vi "FPGA_Array to XY.vi"(7 "Init":bool, 11 "All Random Array":fxp<+/-,32,16>[](array[numeric])) -> (0 "y offset new":i16, 1 "y amp. new":fxp<+,16,0>, 2 "x offset new":i16, 3 "x amp. new":fxp<+,16,0>)   [LabVIEW 2015]
uses:
  Controls/FPGA_Array to XYAO State.ctl
  <vilib>/rvi/Emulation/niFpgaGetClockAttributes.vi
  <vilib>/rvi/Emulation/niFpgaSctlEmulationGetInTimedLoop.vi
  <vilib>/rvi/Emulation/niFpgaEmulationReportErrorSimple.vi
  <vilib>/rvi/Emulation/niFpgaCriticalErrorInLSC.vi
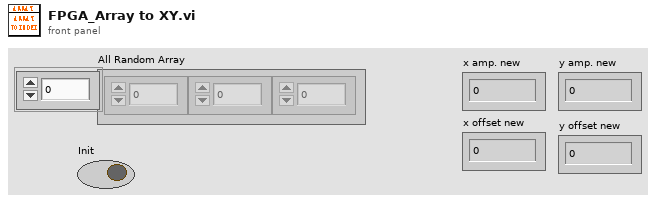
[diagram p1: front panel]
types:
  T1 = typedef "FPGA_Array to XYAO State.ctl" = enum16{"Initial", "Output"}
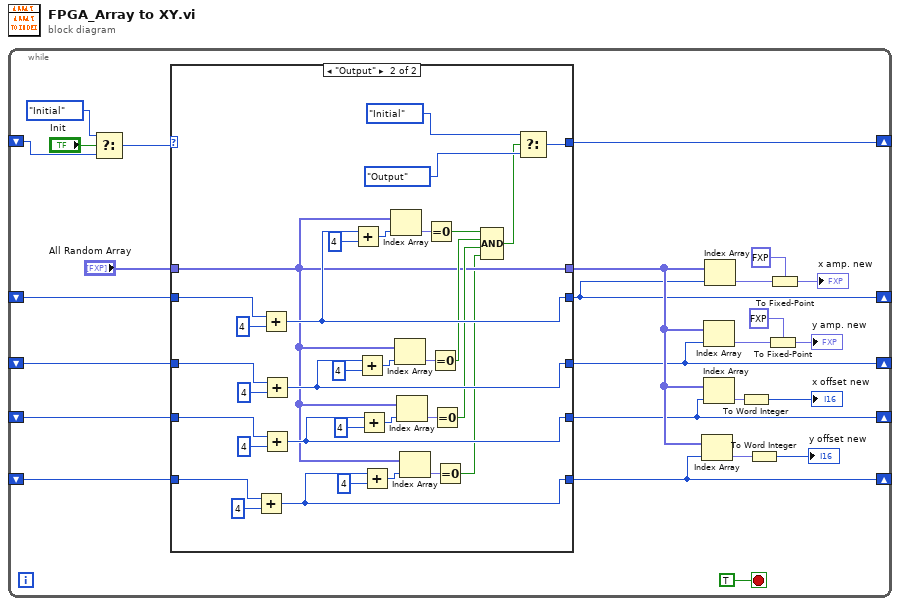
[diagram p0: block diagram]
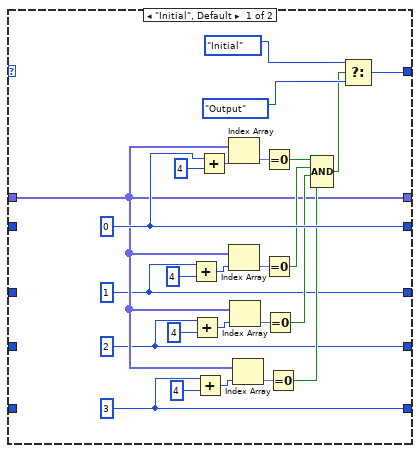
[diagram p2: hidden frame]
diagram:
  n1 = while {
    shift-right: [w12] -> _
    shift-left: _ -> [w25]
    shift-right: [w11] -> _
    shift-left: _ -> [w24]
    shift-right: [w10] -> _
    shift-left: _ -> [w23]
    shift-right: [w9] -> _
    shift-left: _ -> [w22]
    shift-right: [w21] -> _
    shift-left: _ -> [w19]
    stop <- TRUE stop-if-true
    n2 = Select(t=FPGA_Array_to_XYAO_State."Initial" ("Array to XYAO State"), s="Init", f=w19) -> (s? t:f=w20:T1)
    n3 = case shown="\"Output\"" w20 {
      tunnel: w25 -> [_ w84]
      tunnel: w24 -> [_ w81]
      tunnel: w23 -> [_ w80]
      tunnel: w22 -> [_ w77]
      tunnel: [w45 w71] -> w12
      tunnel: [w29 w64] -> w11
      tunnel: [w27 w53] -> w9
      tunnel: [w28 w59] -> w10
      tunnel: [w48 w76] -> w21
      tunnel: "All Random Array" -> [w30 w54]
      tunnel: [w30 w54] -> w13
      frame "Initial", Default {
        w27 = 3
        w28 = 2
        w29 = 1
        w45 = 0
        n4 = Add(x=w29, y=4) -> (x+y=w43:i32)
        n5 = Add(x=w28, y=4) -> (x+y=w37:i32)
        n6 = Add(x=w27, y=4) -> (x+y=w34:i32)
        n7 = Add(x=w45, y=4) -> (x+y=w46:i32)
        n8 = Index Array(array=w30, index=w46) -> (element=w49:fxp<+/-,32,16>)
        n9 = Index Array(array=w30, index=w43) -> (element=w42:fxp<+/-,32,16>)
        n10 = Index Array(array=w30, index=w37) -> (element=w38:fxp<+/-,32,16>)
        n11 = Index Array(array=w30, index=w34) -> (element=w33:fxp<+/-,32,16>)
        n12 = Equal To 0?(x=w49) -> (x = 0?=w40:bool)
        n13 = Equal To 0?(x=w42) -> (x = 0?=w39:bool)
        n14 = Equal To 0?(x=w38) -> (x = 0?=w32:bool)
        n15 = Equal To 0?(x=w33) -> (x = 0?=w31:bool)
        n16 = Compound Arithmetic op=AND ("复合运算")(w40, w39, w32, w31) -> (w41:bool)
        n17 = Select(t=FPGA_Array_to_XYAO_State."Initial" ("Array to XYAO State"), s=w41, f=FPGA_Array_to_XYAO_State."Output" ("Array to XYAO State")) -> (s? t:f=w48:T1)
      }
      frame "Output" {
        n18 = Add(x=w77, y=4) -> (x+y=w53:i32)
        n19 = Add(x=w84, y=4) -> (x+y=w71:i32)
        n20 = Add(x=w81, y=4) -> (x+y=w64:i32)
        n21 = Add(x=w80, y=4) -> (x+y=w59:i32)
        n22 = Add(x=w71, y=4) -> (x+y=w72:i32)
        n23 = Add(x=w64, y=4) -> (x+y=w66:i32)
        n24 = Add(x=w59, y=4) -> (x+y=w61:i32)
        n25 = Add(x=w53, y=4) -> (x+y=w56:i32)
        n26 = Index Array(array=w54, index=w72) -> (element=w73:fxp<+/-,32,16>)
        n27 = Index Array(array=w54, index=w66) -> (element=w65:fxp<+/-,32,16>)
        n28 = Index Array(array=w54, index=w61) -> (element=w62:fxp<+/-,32,16>)
        n29 = Index Array(array=w54, index=w56) -> (element=w55:fxp<+/-,32,16>)
        n30 = Equal To 0?(x=w73) -> (x = 0?=w68:bool)
        n31 = Equal To 0?(x=w65) -> (x = 0?=w63:bool)
        n32 = Equal To 0?(x=w62) -> (x = 0?=w58:bool)
        n33 = Equal To 0?(x=w55) -> (x = 0?=w52:bool)
        n34 = Compound Arithmetic op=AND ("复合运算")(w68, w63, w58, w52) -> (w69:bool)
        n35 = Select(t=FPGA_Array_to_XYAO_State."Initial" ("Array to XYAO State"), s=w69, f=FPGA_Array_to_XYAO_State."Output" ("Array to XYAO State")) -> (s? t:f=w76:T1)
      }
    }
    n36 = Index Array(array=w13, index=w9) -> (element=w16:fxp<+/-,32,16>)
    n37 = Index Array(array=w13, index=w11) -> (element=w5:fxp<+/-,32,16>)
    n38 = Index Array(array=w13, index=w10) -> (element=w3:fxp<+/-,32,16>)
    n39 = Index Array(array=w13, index=w12) -> (element=w15:fxp<+/-,32,16>)
    n40 = To Word Integer(number=w3) -> (16bit integer=→"x offset new":i16)
    n41 = To Word Integer(number=w16) -> (16bit integer=→"y offset new":i16)
    n42 = To Fixed-Point(fixed-point type=fxp<+,16,0> 0.0 ("x amp. new"), number=w5) -> (fixed-point=→"y amp. new":fxp<+,16,0>)
    n43 = To Fixed-Point(fixed-point type=fxp<+,16,0> 0.0 ("x amp. new"), number=w15) -> (fixed-point=→"x amp. new":fxp<+,16,0>)
  }
